vi "Excel_Insert_Chart.vi"(0 "AddOLEObject":refnum<k7>, 1 "Excel._Worksheet":refnum<k7>, 5 "column header":string[](array[string]), 7 "row header":string[](array[string]), 9 "Data":dbl[][](array[numeric]) format="%0.2f", 11 "error in (no error)":errorcluster, 12 "ChartType":i32(ring)=51 items=["xlColumnClustered"=51, "xlColumnStacked"=52, "xlColumnStacked100"=53, "xl3DColumnClustered"=54, "xl3DColumnStacked"=55, "xl3DColumnStacked100"=56, "xlBarClustered"=57, "xlBarStacked"=58, "xlBarStacked100"=59, "xl3DBarClustered"=60, "xl3DBarStacked"=61, "xl3DBarStacked100"=62, "xlLineStacked"=63, "xlLineStacked100"=64, "xlLineMarkers"=65, "xlLineMarkersStacked"=66, "xlLineMarkersStacked100"=67, "xlPieOfPie"=68, "xlPieExploded"=69, "xl3DPieExploded"=70, "xlBarOfPie"=71, "xlXYScatterSmooth"=72, "xlXYScatterSmoothNoMarkers"=73, "xlXYScatterLines"=74, "xlXYScatterLinesNoMarkers"=75, "xlAreaStacked"=76, "xlAreaStacked100"=77, "xl3DAreaStacked"=78, "xl3DAreaStacked100"=79, "xlDoughnutExploded"=80, "xlRadarMarkers"=81, "xlRadarFilled"=82, "xlSurface"=83, "xlSurfaceWireframe"=84, "xlSurfaceTopView"=85, "xlSurfaceTopViewWireframe"=86, "xlBubble"=15, "xlBubble3DEffect"=87, "xlStockHLC"=88, "xlStockOHLC"=89, "xlStockVHLC"=90, "xlStockVOHLC"=91, "xlCylinderColClustered"=92, "xlCylinderColStacked"=93, "xlCylinderColStacked100"=94, "xlCylinderBarClustered"=95, "xlCylinderBarStacked"=96, "xlCylinderBarStacked100"=97, "xlCylinderCol"=98, "xlConeColClustered"=99, "xlConeColStacked"=100, "xlConeColStacked100"=101, "xlConeBarClustered"=102, "xlConeBarStacked"=103, "xlConeBarStacked100"=104, "xlConeCol"=105, "xlPyramidColClustered"=106, "xlPyramidColStacked"=107, "xlPyramidColStacked100"=108, "xlPyramidBarClustered"=109, "xlPyramidBarStacked"=110, "xlPyramidBarStacked100"=111, "xlPyramidCol"=112, "xl3DColumn"=-4100, "xlLine"=4, "xl3DLine"=-4101, "xl3DPie"=-4102, "xlPie"=5, "xlXYScatter"=-4169, "xl3DArea"=-4098, "xlArea"=1, "xlDoughnut"=-4120, "xlRadar"=-4151], 13 "Chart title":string, 14 "has legend?":bool) -> (15 "error out":errorcluster)   [LabVIEW 2010, in "NI_ReportGenerationToolkit.lvlib"]
doc: "This VI opens Excel by creating an Automation Refnum for the Excel.Application object. Next it sets the \"Visible\" property to True/False depending on the Visible input."
uses:
  <vilib>/addons/_office/NI_ReportGenerationToolkit.lvlib
  <vilib>/Utility/NIReport.llb/NI_ReportGenerationCore.lvlib
panel:
  in  "Graph.Chart":refnum<k7>
  in  "Excel._OLEObject":refnum<k7>
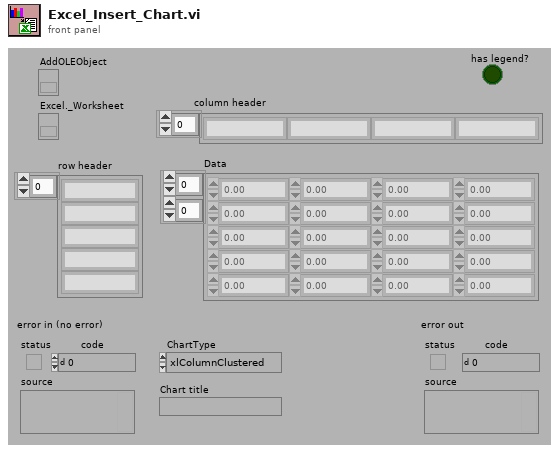
[diagram p1: front panel]
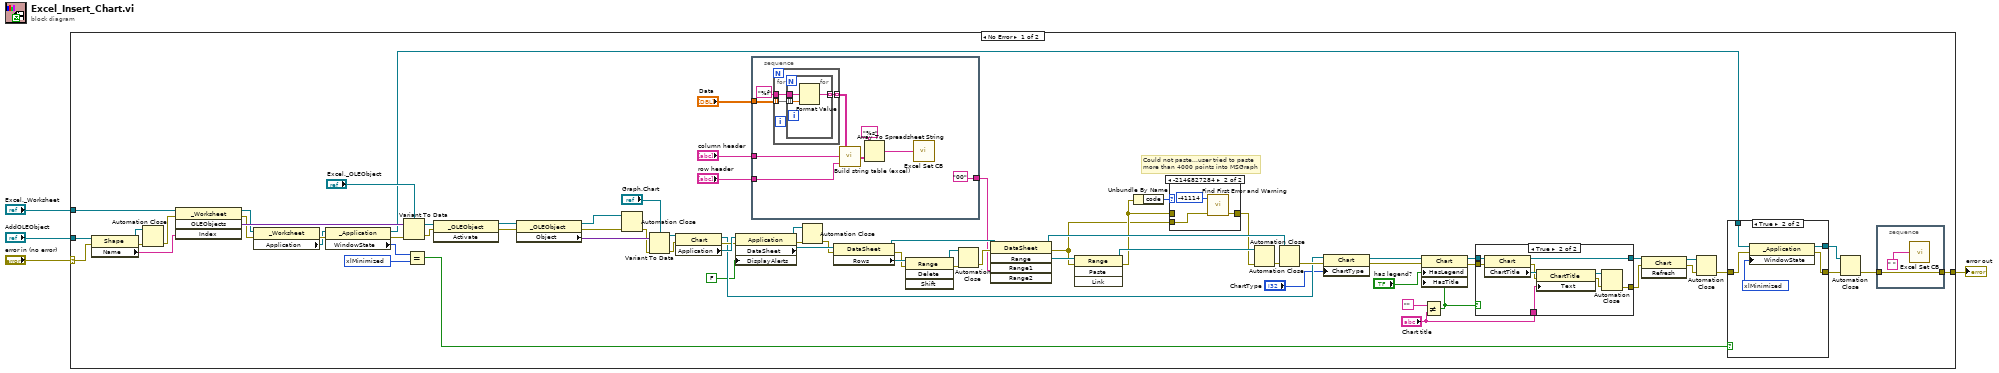
[diagram p0: block diagram]
diagram:
  n1 = case shown="No Error" "error in (no error)" {
    selector: "error in (no error)" -> [w6 w118]
    tunnel: "AddOLEObject" -> [w39 _]
    tunnel: [w36 w118] -> w3
    tunnel: "Excel._Worksheet" -> [w21 _]
    frame No Error {
      w17 = -4140 items=["xlMaximized"=-4137, "xlMinimized"=-4140, "xlNormal"=-4143] ("WindowState")
      # "Could not paste...user tried to paste\nmore than 4000 points into MSGraph"
      n2 = property class="Shape"(reference=w39, error in=w6) -> (reference out=w77:refnum<k7>, error out=w78:errorcluster, "Name"=w76:string)
      n3 = Automation Close(3:w78, 5:w77) -> (0:w75:errorcluster)
      n4 = invoke class="_Worksheet" method="OLEObjects"(reference=w21, error in=w75, "Index"=w76) -> (reference out=w26:refnum<k7>, error out=w25:errorcluster, "OLEObjects"=w71:variant)  [unwired: 1 in, 1 out]
      n5 = property class="_Worksheet"(reference=w26, error in=w25) -> (error out=w24:errorcluster, "Application"=w20:refnum<k7>)  [unwired: 1 out]
      n6 = property class="_Application"(reference=w20, error in=w24) -> (reference out=w14:refnum<k7>, error out=w19:errorcluster, "WindowState"=w18:i32)
      n7 = Variant To Data(error in=w19, Variant=w71, type="Excel._OLEObject") -> (error out=w29:errorcluster, data=w28:refnum<k7>)
      n8 = Equal?(x=w18, y=w17) -> (x = y?=w16:bool)
      n9 = invoke class="_OLEObject" method="Activate"(reference=w28, error in=w29) -> (reference out=w27:refnum<k7>, error out=w30:errorcluster)  [unwired: 1 in, 1 out]
      n10 = property class="_OLEObject"(reference=w27, error in=w30) -> (reference out=w43:refnum<k7>, error out=w62:errorcluster, "Object"=w72:variant)
      n11 = Automation Close(3:w62, 5:w43) -> (0:w61:errorcluster)
      n12 = Variant To Data(error in=w61, Variant=w72, type="Graph.Chart") -> (error out=w51:errorcluster, data=w45:refnum<k7>)
      n13 = property class="Chart"(reference=w45, error in=w51) -> (reference out=w42:refnum<k7>, error out=w44:errorcluster, "Application"=w60:refnum<k7>)
      n14 = property class="Application"(reference=w60, error in=w44, "DisplayAlerts"=FALSE) -> (reference out=w22:refnum<k7>, error out=w38:errorcluster, "DataSheet"=w41:refnum<k7>)
      n15 = stacked-sequence {
        tunnel: "Data" -> [w98]
        tunnel: "row header" -> [w97]
        tunnel: "column header" -> [w96]
        tunnel: ["00"] -> w46
        frame #0 {
          n16 = for {
            tunnel: w98 -> [w101] mode=indexing
            tunnel: "%f" -> [w100]
            tunnel: [w99] -> w94 mode=indexing
            n17 = for {
              tunnel: w101 -> [w104] mode=indexing
              tunnel: w100 -> [w103]
              tunnel: [w102] -> w99 mode=indexing
              n18 = Format Value(format string=w103, value (0)=w104) -> (output string=w102:string)  [unwired: 1 out]
            }
          }
          n19 = call <vilib>:"Build string table (excel).vi"("row headers"=w97, "column headers"=w96, "text data"=w94) -> ("output table"=w92:string[][])
          n20 = Array To Spreadsheet String(array=w92, 3:"%s" ("format string")) -> (spreadsheet string=w90:string)  [unwired: 1 out]
          n21 = call <vilib>:"Excel Set CB.vi"("String"=w90) -> ()  [unwired: 1 out]
        }
      }
      n22 = Automation Close(3:w38, 5:w22) -> (0:w37:errorcluster)
      n23 = property class="DataSheet"(reference=w41, error in=w37) -> (reference out=w56:refnum<k7>, error out=w54:errorcluster, "Rows"=w55:refnum<k7>)
      n24 = invoke class="Range" method="Delete"(reference=w55, error in=w54) -> (reference out=w52:refnum<k7>, error out=w53:errorcluster)  [unwired: 2 in, 2 out]
      n25 = Automation Close(3:w53, 5:w52) -> (0:w58:errorcluster)
      n26 = invoke class="DataSheet" method="Range"(reference=w56, error in=w58, "Range1"=w46) -> (reference out=w40:refnum<k7>, error out=w7:errorcluster, "Range"=w57:refnum<k7>)  [unwired: 2 in, 2 out]
      n27 = invoke class="Range" method="Paste"(reference=w57, error in=w7) -> (reference out=w23:refnum<k7>, error out=w9:errorcluster)  [unwired: 2 in, 2 out]
      n28 = Unbundle By Name(w9) -> ("code"=w10:i32)
      n29 = case shown="-2146827284" w10 {
        tunnel: w9 -> [w79 _]
        tunnel: [w79 w82] -> w8
        tunnel: w7 -> [_ w80]
        frame Default {
        }
        frame -2146827284 {
          n30 = call <vilib>:"Find First Error and Warning.vi"("error in (no error)"=w80, "error code"=-41114) -> ("error out"=w82:errorcluster)  [unwired: 5 out]
        }
      }
      n31 = Automation Close(3:w8, 5:w23) -> (0:w59:errorcluster)
      n32 = Automation Close(3:w59, 5:w40) -> (0:w50:errorcluster)
      n33 = property class="Chart"(reference=w42, error in=w50, "ChartType"="ChartType") -> (reference out=w70:refnum<k7>, error out=w69:errorcluster)
      n34 = Not Equal?(x="", y="Chart title") -> (x != y?=w64:bool)
      n35 = property class="Chart"(reference=w70, error in=w69, "HasLegend"="has legend?", "HasTitle"=w64) -> (reference out=w68:refnum<k7>, error out=w67:errorcluster)
      n36 = case shown="True" w64 {
        tunnel: w68 -> [w107 w117]
        tunnel: w67 -> [w108 w115]
        tunnel: [w108 w111] -> w32
        tunnel: "Chart title" -> [_ w110]
        tunnel: [w107 w109] -> w34
        frame False {
        }
        frame True {
          n37 = property class="Chart"(reference=w117, error in=w115) -> (reference out=w109:refnum<k7>, error out=w114:errorcluster, "ChartTitle"=w116:refnum<k7>)
          n38 = property class="ChartTitle"(reference=w116, error in=w114, "Text"=w110) -> (reference out=w113:refnum<k7>, error out=w112:errorcluster)
          n39 = Automation Close(3:w112, 5:w113) -> (0:w111:errorcluster)
        }
      }
      n40 = invoke class="Chart" method="Refresh"(reference=w34, error in=w32) -> (reference out=w33:refnum<k7>, error out=w31:errorcluster)  [unwired: 1 in, 1 out]
      n41 = Automation Close(3:w31, 5:w33) -> (0:w15:errorcluster)
      n42 = case shown="True" w16 {
        tunnel: w15 -> [w84 w88]
        tunnel: w14 -> [w83 w87]
        tunnel: [w84 w86] -> w13
        tunnel: [w83 w85] -> w11
        frame False {
        }
        frame True {
          w89 = -4140 items=["xlMaximized"=-4137, "xlMinimized"=-4140, "xlNormal"=-4143] ("WindowState")
          n43 = property class="_Application"(reference=w87, error in=w88, "WindowState"=w89) -> (reference out=w85:refnum<k7>, error out=w86:errorcluster)
        }
      }
      n44 = Automation Close(3:w13, 5:w11) -> (0:w12:errorcluster)
      n45 = stacked-sequence {
        tunnel: w12 -> [w106]
        tunnel: [w106] -> w36
        frame #0 {
          n46 = call <vilib>:"Excel Set CB.vi"("String"=" ") -> ()  [unwired: 1 out]
        }
      }
    }
    frame Error {
    }
  }
  "error out" <- w3
